vi "create.vi"(8 "error in (no error)":errorcluster, 11 "path":path) -> (0 "error out":errorcluster, 3 "logging":refnum<class "system.logging.lvclass">)   [LabVIEW 2021, in "system.logging.lvclass"]
uses:
  system.logging.lvclass
  system.logging.lvclass/system.logging.ctl
panel:
  # "Create the logger and add it to the system container."
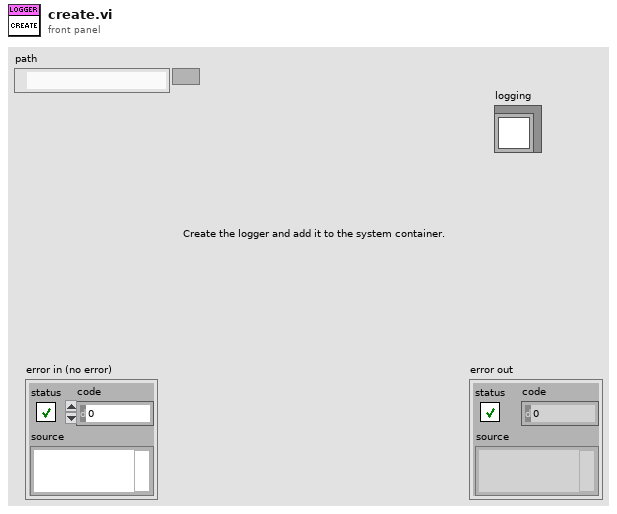
[diagram p1: front panel]
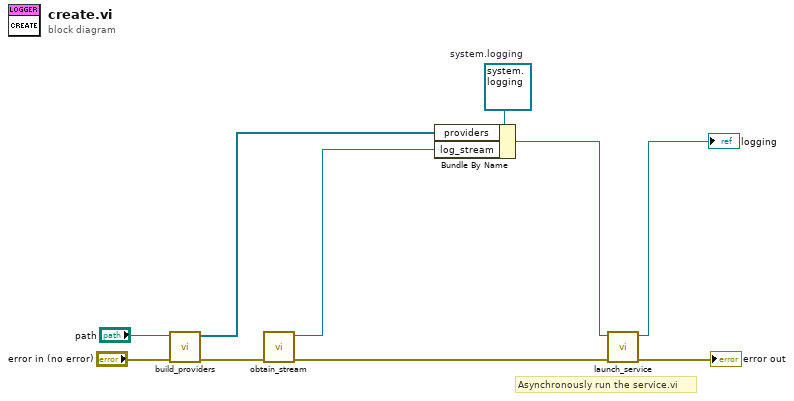
[diagram p0: block diagram]
diagram:
  w10 = refnum<class "system.logging.lvclass"> refnum  # system.logging
  # "Asynchronously run the service.vi"
  n1 = call "build_providers.vi"("error in"="error in (no error)", "path"="path") -> ("error out"=w8:errorcluster, "providers"=w7:refnum<class "system.logging.provider.lvclass">[])  [unwired: 8 in]
  n2 = call "obtain_stream.vi"("error in (no error)"=w8) -> ("error out"=w2:errorcluster, "log_stream"=w1:refnum<queue>)  [unwired: 9 in]
  n3 = Bundle By Name(cluster=w10, "providers"=w7, "log_stream"=w1) -> (w4:refnum<class "system.logging.lvclass">)
  n4 = call "launch_service.vi"("error in (no error)"=w2, "system.logging in"=w4) -> ("error out"=→"error out":errorcluster, "system.logging out"=→"logging":refnum<class "system.logging.lvclass">)  [unwired: 8 in]
